vi "number_to_switches.vi"(4 "error in (no error)":errorcluster, 7 "number":u8) -> (0 "error out":errorcluster, 3 "switches":bool[](array[boolean]))   [LabVIEW 2018]
doc: "convertes a number (the 'data') to a bollean array with 8 switches to a number."
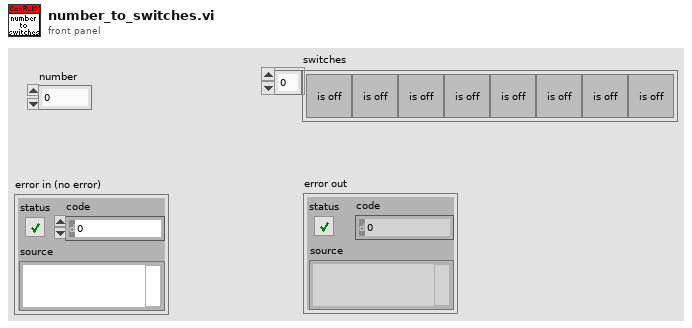
[diagram p1: front panel]
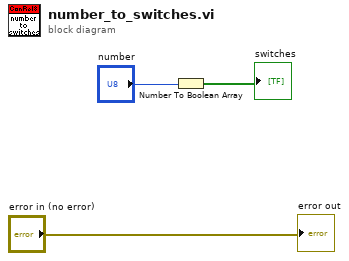
[diagram p0: block diagram]
diagram:
  n1 = Number To Boolean Array(number="number") -> (Boolean array=→"switches":bool[])
  "error out" <- "error in (no error)"
